vi "util_launch_step_action.vi"(5 "waitgroup":T4, 7 "references":T1, 8 "error in (no error)":errorcluster, 10 "data":variant, 11 "step_vi_reference":T3) -> (0 "error out":errorcluster)   [LabVIEW 2015, in "lv-recipe-machine.lvlib"]
uses:
  lv-recipe-machine.lvlib
  <userlib>/antonio-alexander/lv-waitgroup/public/_controls/api_waitgroup.ctl
  public/_controls/step_vi_reference.ctl
  public/_controls/references.ctl
  _controls/input.ctl
  _controls/input_command.ctl
  _controls/output.ctl
  _controls/data.ctl
  public/_controls/configuration.ctl
  _controls/recipe_data.ctl
  public/_controls/mode.ctl
  public/_controls/manual_state.ctl
  public/_controls/automatic_state.ctl
  public/_controls/recipe_step.ctl
  public/_controls/transition.ctl
  public/_controls/change.ctl
  public/_controls/status.ctl
  public/_controls/step_references.ctl
  <userlib>/antonio-alexander/lv-waitgroup/lv-waitgroup.lvlib
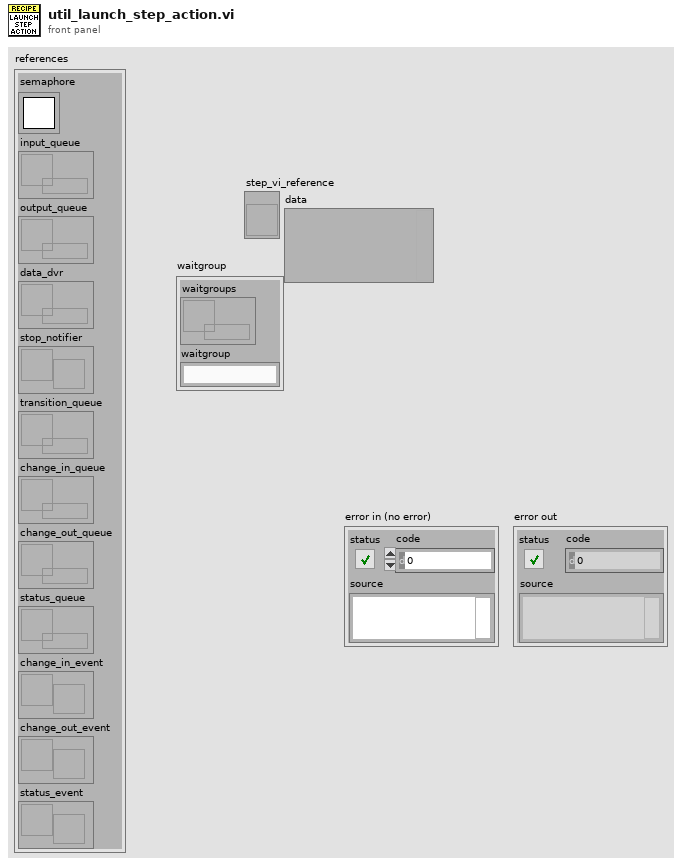
[diagram p1: front panel]
types:
  T1 = typedef "lv-recipe-machine.lvlib/references.ctl" = cluster{"semaphore":T2, "input_queue":refnum<queue>, "output_queue":refnum<queue>, "data_dvr":refnum<data-value>, "stop_notifier":refnum<notifier>, "transition_queue":refnum<queue>, "change_in_queue":refnum<queue>, "change_out_queue":refnum<queue>, "status_queue":refnum<queue>, "change_in_event":refnum<user-event>, "change_out_event":refnum<user-event>, "status_event":refnum<user-event>}
  T2 = typedef "Semaphore RefNum" = refnum<k1>
  T3 = typedef "lv-recipe-machine.lvlib/step_vi_reference.ctl" = refnum<vi>
  T4 = typedef "lv-waitgroup.lvlib/api_waitgroup.ctl" = cluster{"waitgroups":refnum<data-value>, "waitgroup":string}
  T5 = typedef "lv-recipe-machine.lvlib/step_references.ctl" = cluster{"references":T1, "api_waitgroup":T4}
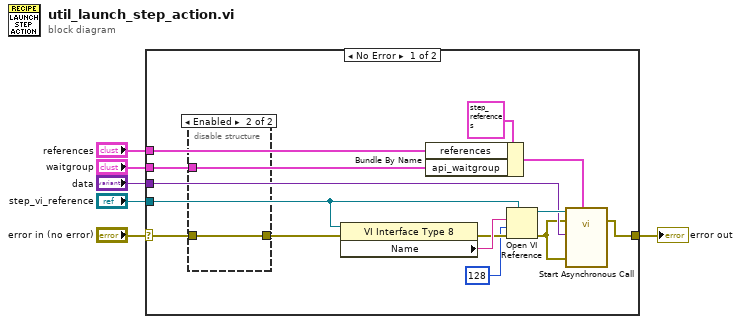
[diagram p0: block diagram]
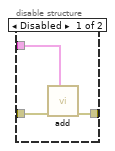
[diagram p2: hidden frame]
diagram:
  n1 = case shown="No Error" "error in (no error)" {
    selector: "error in (no error)" -> [w15 w25]
    tunnel: "waitgroup" -> [w10 _]
    tunnel: [w14 w25] -> w4
    tunnel: "step_vi_reference" -> [w13 _]
    tunnel: "data" -> [w12 _]
    tunnel: "references" -> [w9 _]
    frame No Error {
      n2 = disable-structure shown="Enabled" {
        disable-tunnel: [w23 w24] -> w20
        disable-tunnel: w15 -> [w22 w24]
        disable-tunnel: w10 -> [w21 _]
        frame Disabled {
          n3 = call <userlib>:"add.vi"("waitgroup"=w21, "error in (no error)"=w22) -> ("error out"=w23:errorcluster)  [unwired: 9 in]
        }
        frame Enabled {
        }
      }
      n4 = property class="VI Interface Type 8"(reference=w13, error in=w20) -> (error out=w18:errorcluster, "Name"=w19:string)  [unwired: 1 out]
      n5 = Bundle By Name(cluster=T5 {"references"={"semaphore"=refnum, "input_queue"=refnum, "output_queue"=refnum, "data_dvr"=refnum, "stop_notifier"=refnum, "transition_queue"=refnum, "change_in_queue"=refnum, "change_out_queue"=refnum, "status_queue"=refnum, "change_in_event"=refnum, "change_out_event"=refnum, "status_event"=refnum}, "api_waitgroup"={"waitgroups"=refnum, "waitgroup"=""}} ("step_references"), "references"=w9, "api_waitgroup"=w10) -> (w7:T5)
      n6 = Open VI Reference(type specifier VI Refnum (for type only)=w13, vi path=w19, options=128, error in (no error)=w18) -> (vi reference=w17:T3, error out=w11:errorcluster)  [unwired: 2 in]
      n7 = call-by-ref "Start Asynchronous Call"(reference=w17, error in=w11, "step_references"=w7, 8:"error in (no error)"=w11, "data"=w12) -> (error out=w14:errorcluster)  [unwired: 8 in, 2 out]
    }
    frame Error {
    }
  }
  "error out" <- w4
